vi "upload_file.vi"(8 "error in (no error)":errorcluster, 9 "portal_upload_path":string="skynet/skyfile", 10 "portal_url":string="https://siasky.net/", 11 "Local File Path":path=path "D:/") -> (0 "error out":errorcluster, 3 "skylink":string)   [LabVIEW 2019, in "SiaSkynetAPI.lvlib"]
uses:
  SiaSkynetAPI.lvlib
  <vilib>/httpClient/MultipartData.ctl
  <vilib>/httpClient/LabVIEWHTTPClient.lvlib
panel:
  out "body":string
  out "headers":string
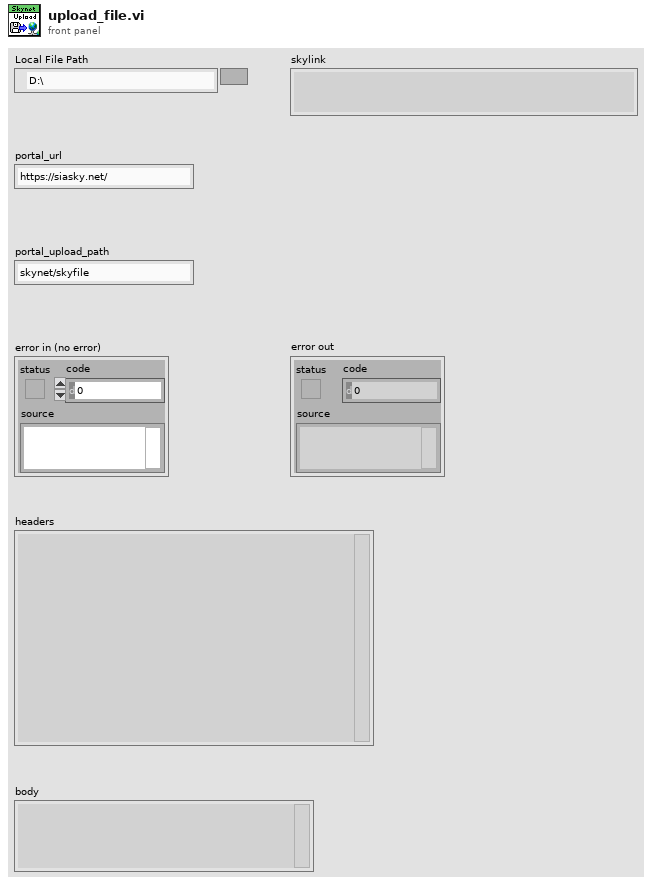
[diagram p1: front panel]
types:
  T1 = typedef "LabVIEWHTTPClient.lvlib/MultipartData.ctl" = cluster{"Name":string, "Value":string, "File":path, "Filename":string, "MIME type":string}
  T2 = typedef "LabVIEWHTTPClient.lvlib/ClientHandle.ctl" = refnum<k1>
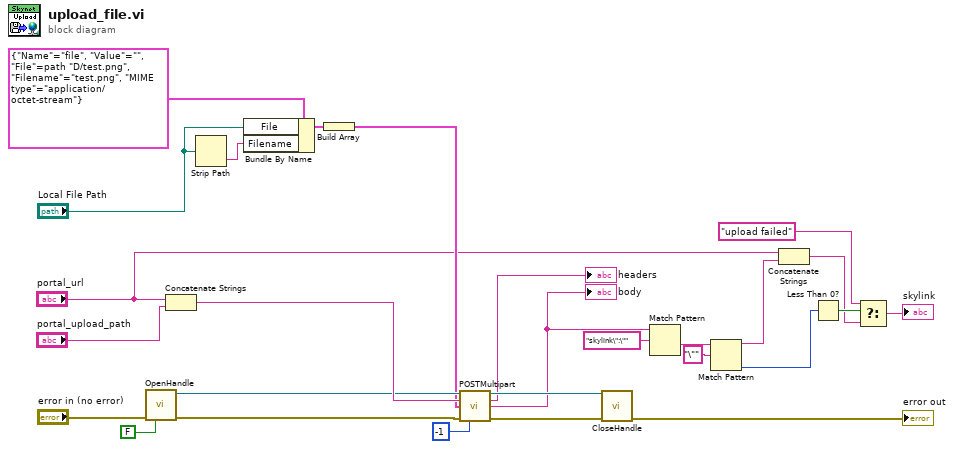
[diagram p0: block diagram]
diagram:
  n1 = call <vilib>:"OpenHandle.vi"("error in (no error)"="error in (no error)", "verify server(true)"=FALSE) -> ("client handle out"=w21:T2, "error out"=w20:errorcluster)  [unwired: 12 in]
  n2 = Concatenate Strings("portal_url", "portal_upload_path") -> (w22:string)
  n3 = Strip Path(path="Local File Path") -> (name=w13:string)  [unwired: 1 out]
  n4 = Bundle By Name(cluster=T1 {"Name"="file", "Value"="", "File"=path "D:/test.png", "Filename"="test.png", "MIME type"="application/octet-stream"} ("Element"), "File"="Local File Path", "Filename"=w13) -> (w16:T1)
  n5 = Build Array(w16) -> (w15:T1[])
  n6 = call <vilib>:"POSTMultipart.vi"("client handle"=w21, "url"=w22, "data"=w15, "error in (no error)"=w20, "timeout (10000)"=-1) -> ("client handle out"=w27:T2, "headers"=→"headers":string, "body"=w12:string, "error out"=w26:errorcluster)  [unwired: 7 in]
  "body" <- w12
  n7 = call <vilib>:"CloseHandle.vi"("client handle"=w27, "error in (no error)"=w26) -> ("error out"=→"error out":errorcluster)  [unwired: 13 in]
  n8 = Match Pattern(string=w12, regular expression="skylink\":\"") -> (after substring=w10:string)  [unwired: 1 in, 3 out]
  n9 = Match Pattern(string=w10, regular expression="\"") -> (before substring=w7:string, offset past match=w5:i32)  [unwired: 1 in, 2 out]
  n10 = Concatenate Strings("portal_url", w7) -> (w4:string)
  n11 = Less Than 0?(x=w5) -> (x < 0?=w6:bool)
  n12 = Select(t="upload failed", s=w6, f=w4) -> (s? t:f=→"skylink":string)
